vi "IsHttpUrl.vi"(8 "Error In":errorcluster, 11 "URL":string="https://download.ni.com/support/nipkg/products/ni-t/ni-teststand-2020/20.0/released") -> (0 "Error Out":errorcluster, 3 "Web URL?":bool)   [LabVIEW 2019, in "CEPM.lvlib"]
uses:
  CEPM.lvlib
  <vilib>/regexp/Match Regular Expression.xnode
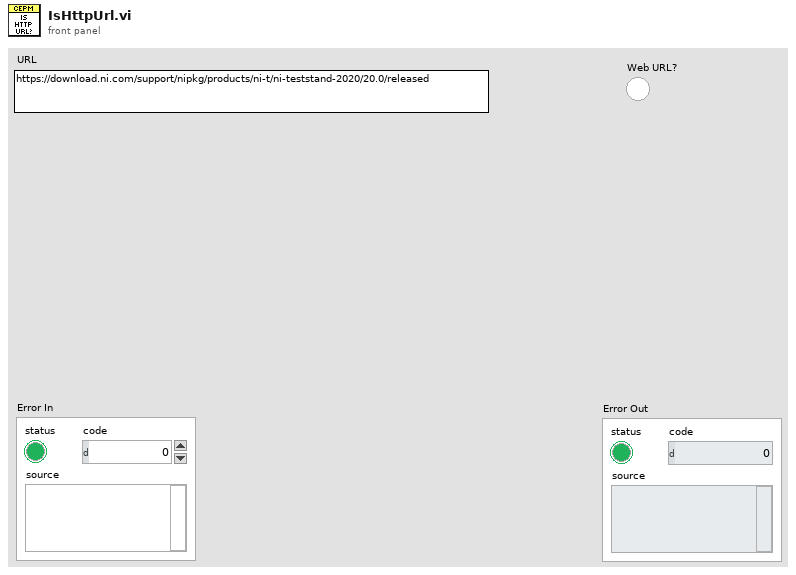
[diagram p1: front panel]
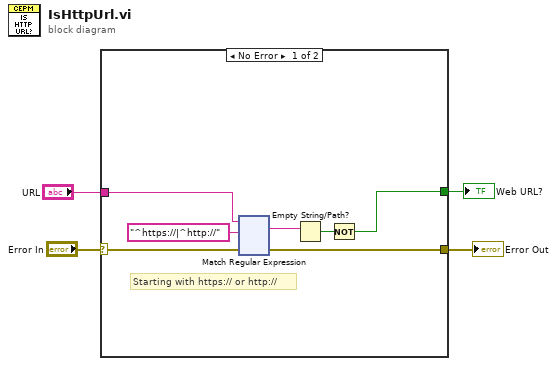
[diagram p0: block diagram]
diagram:
  n1 = case shown="No Error" "Error In" {
    selector: "Error In" -> [w11 w126]
    tunnel: [w5 w126] -> w3
    tunnel: "URL" -> [w10 _]
    tunnel: [w6 _] -> w1
    frame No Error {
      # "Starting with https:// or http://"
      n2 = xnode "Match Regular Expression"("input string"=w10, "regular expression"="^https://|^http://", "error in"=w11) -> ("whole match"=w8:string, "error out"=w5:errorcluster)  [unwired: 3 in, 3 out]
      n3 = Empty String/Path?(string/path=w8) -> (empty?=w7:bool)
      n4 = Not(x=w7) -> (.not. x?=w6:bool)
    }
    frame Error {
    }
  }
  "Error Out" <- w3
  "Web URL?" <- w1
